vi "OE1022_Configure Equation.vi"(7 "OE1022_Configure Equation":T1={"A"=0, "B"=18, "C"=19, "E"=1, "C1"=0.0, "C2"=0.0} {"C2" min=-10.0 max=10.0 format="%.3f"; "C1" min=-10.0 max=10.0 format="%.3f"; "E" items=["1"=1, "2"=2, "3"=3, "4"=4]; "C" items=["R", "X", "Y", "Theta", "Rh1", "Xh1", "Yh1", "Theta h1", "Rh2", "Xh2", "Yh2", "Theta h2", "Noise", "A1", "A2", "A3", "A4", "Freq", "C1", "C2"]; "B" items=["R", "X", "Y", "Theta", "Rh1", "Xh1", "Yh1", "Theta h1", "Rh2", "Xh2", "Yh2", "Theta h2", "Noise", "A1", "A2", "A3", "A4", "Freq", "C1", "C2"]; "A" items=["R", "X", "Y", "Theta", "Rh1", "Xh1", "Yh1", "Theta h1", "Rh2", "Xh2", "Yh2", "Theta h2", "Noise", "A1", "A2", "A3", "A4", "Freq", "C1", "C2"]}, 8 "Error in (no error)":errorcluster caption="error out（no error）", 9 "Remote Mode":u16(ring) items=["USB"=0, "GPIB"=2], 11 "VISA resource name":refnum<visa-resource-name>) -> (0 "Error out":errorcluster caption="error out", 1 "Output String":string, 3 "VISA resource  out":refnum<visa-resource-name>)   [LabVIEW 2011]
panel:
  # "X"
  # "="
  # "______________________________________________________"
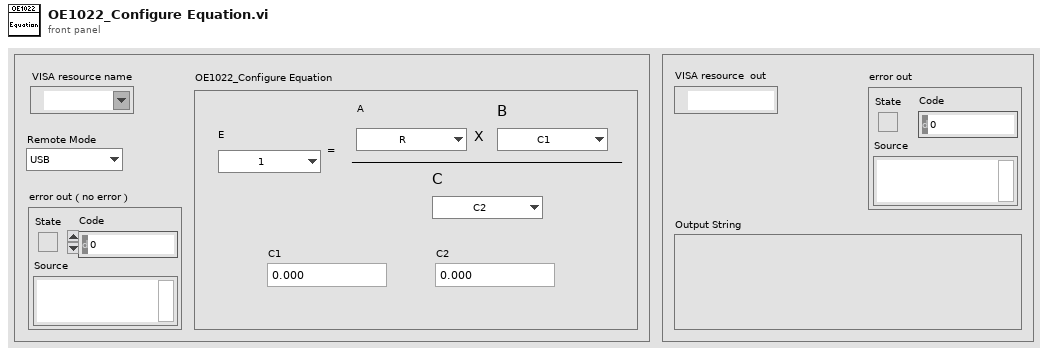
[diagram p1: front panel]
types:
  T1 = cluster{"A":u16, "B":u16, "C":u16, "E":u16, "C1":dbl, "C2":dbl}
  T2 = enum16{"ISRC", "IGND", "ICPL", "ILIN", "PHAS", "FMOD", "RSLP", "FREQ", "SWPT", "SLLM", "SULM", "SSLL", "SSLG", "STLM", "SWRM", "IRNG", "SENS", "RMOD", "OFLT", "OFSL", "SYNC", "DMOD", "HARM", "DARB", "SWVT", "SLVL", "SVLL", "SVUL", "SVSL", "SVSG", "SVTM", "SVRM", "RALL", "SNAP", "OUTP", "OAUX", "COUT", "CAUX", "COFP", "CEXP", "FPOP", "OEXP", "*IDN", "*RST", "OVLD", "INOV", "GNOV", "*PLL", "SSET", "RSET", "AGAN", "APHS", "ARSV", "ASCL", "EQCD", "EQCS", "SPED", "SRAT", "SLEN", "SSLE", "STRG", "SPRM", "STRD", "PAUS", "REST", "SPTS", "TRCA", "TEMP", "RSTU", "IHNZ", "DEQU", "SADD", "ARNG", "CSPE", "ISRCD", "IGNDD", "ICPLD", "ILIND", "PHASD", "FMODD", "RSLPD", "FREQD", "SWPTD", "SLLMD", "SULMD", "SSLLD", "SSLGD", "STLMD", "SWRMD", "SENSD", "RMODD", "OFLTD", "OFSLD", "SYNCD", "HARMD", "EQCDD", "EQCSD", "SNAPD", "OUTPD", "SWVTD", "SLVLD", "SVLLD", "SVULD", "SVSLD", "SVSGD", "SVTMD", "SVRMD", "SVDCD", "ARSVD", "AGAND", "APHSD", "ASCLD", "FPOPD", "CAUXD", "OEXPD", "SPEDD", "SRATD", "SLEND", "SSLED", "STRGD", "SPRMD", "STRDD", "PAUSD", "RESTD", "SPTSD", "TRCAD", "*IDND", "*RSTD", "INOVD", "GNOVD", "*PLLD", "SSETD", "RSETD"}
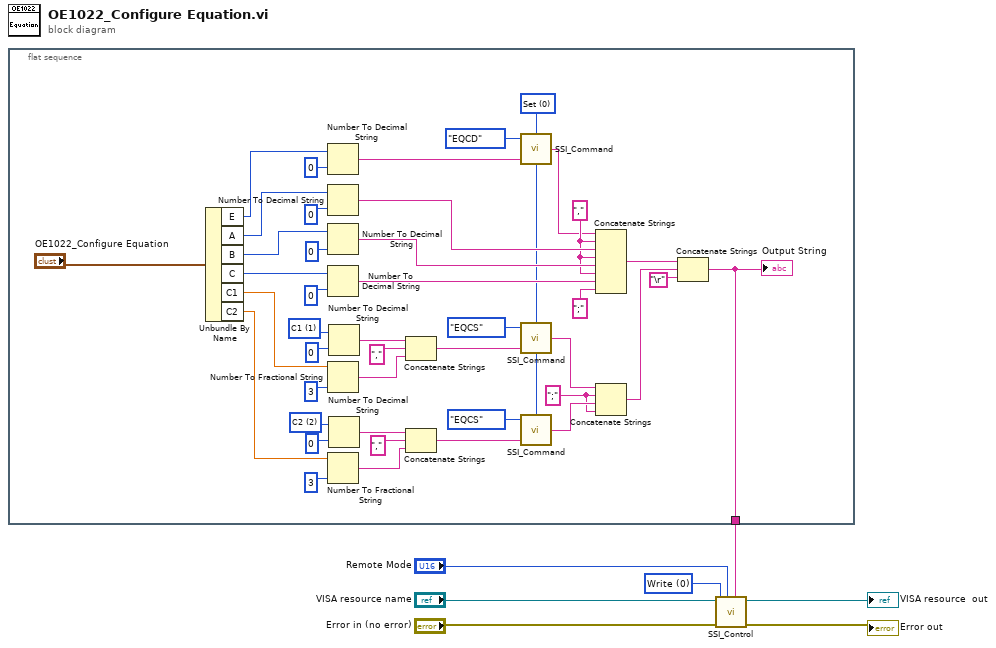
[diagram p0: block diagram]
diagram:
  w6 = u16 0 items=["Write", "Read"] ("Control")
  n1 = flat-sequence {
    tunnel: [w48] -> w1
    frame #0 {
      w12 = ";" ("替换字符串(\"\")")
      w21 = u16 0 items=["Set", "Query"] ("Opera")
      w23 = u16 2 items=["C1"=1, "C2"=2]
      w24 = u16 1 items=["C1"=1, "C2"=2]
      w31 = "," ("替换字符串(\"\")")
      n2 = Unbundle By Name("OE1022_Configure Equation") -> ("E"=w38:u16, "A"=w37:u16, "B"=w36:u16, "C"=w35:u16, "C1"=w9:dbl, "C2"=w8:dbl)
      n3 = Number To Decimal String(number=w38, width (-)=i16 0 ("精度(6)")) -> (decimal integer string=w11:string)
      n4 = Number To Decimal String(number=w37, width (-)=i16 0 ("宽度(-)")) -> (decimal integer string=w34:string)
      n5 = Number To Decimal String(number=w36, width (-)=i16 0 ("宽度(-)")) -> (decimal integer string=w33:string)
      n6 = Number To Decimal String(number=w35, width (-)=i16 0 ("宽度(-)")) -> (decimal integer string=w32:string)
      n7 = Number To Fractional String(number=w9, precision (6)=i16 3 ("宽度(-)")) -> (F-format string=w18:string)  [unwired: 2 in]
      n8 = Number To Fractional String(number=w8, precision (6)=i16 3 ("宽度(-)")) -> (F-format string=w16:string)  [unwired: 2 in]
      n9 = Number To Decimal String(number=w24, width (-)=i16 0 ("宽度(-)")) -> (decimal integer string=w19:string)
      n10 = Number To Decimal String(number=w23, width (-)=i16 0 ("宽度(-)")) -> (decimal integer string=w17:string)
      n11 = Concatenate Strings(w19, "," ("替换字符串(\"\")"), w18) -> (w20:string)
      n12 = Concatenate Strings(w17, "," ("替换字符串(\"\")"), w16) -> (w15:string)
      n13 = call "SSI_Command.vi"("Opera"=w21, "Paramter"=w11, "Command Type"=T2."EQCD") -> ("Output string"=w10:string)  [unwired: 1 in]
      n14 = call "SSI_Command.vi"("Opera"=w21, "Paramter"=w20, "Command Type"=T2."EQCS") -> ("Output string"=w46:string)  [unwired: 1 in]
      n15 = call "SSI_Command.vi"("Opera"=w21, "Paramter"=w15, "Command Type"=T2."EQCS") -> ("Output string"=w22:string)  [unwired: 1 in]
      n16 = Concatenate Strings(w10, w31, w34, w31, w33, w31, w32, ";" ("替换字符串(\"\")")) -> (w40:string)
      n17 = Concatenate Strings(w46, w12, w22, w12) -> (w28:string)
      n18 = Concatenate Strings(w40, w28, "\r") -> (w48:string)
      "Output String" <- w48
    }
  }
  n19 = call "SSI_Control.vi"("Write Buffer"=w1, "Remote Mode"="Remote Mode", "Error in (no error)"="Error in (no error)", "Control"=w6, "VISA resource name"="VISA resource name") -> ("Error out"=→"Error out":errorcluster, "VISA resource  out"=→"VISA resource  out":refnum<visa-resource-name>)  [unwired: 3 in, 2 out]
